vi "Save VI.vi"(8 "error in (no error)":errorcluster, 10 "Ctl Properties":T1[](array[typedef]), 11 "VI Properties":T2) -> (0 "error out":errorcluster, 2 "Status":bool, 3 "VI out":refnum<vi>)   [LabVIEW 2023, in "VI Properties Editor.lvlib"]
uses:
  VI Properties Editor.lvlib
  VI Properties.ctl
  <vilib>/picture/picture.llb/imagedata.ctl
  Control Properties.ctl
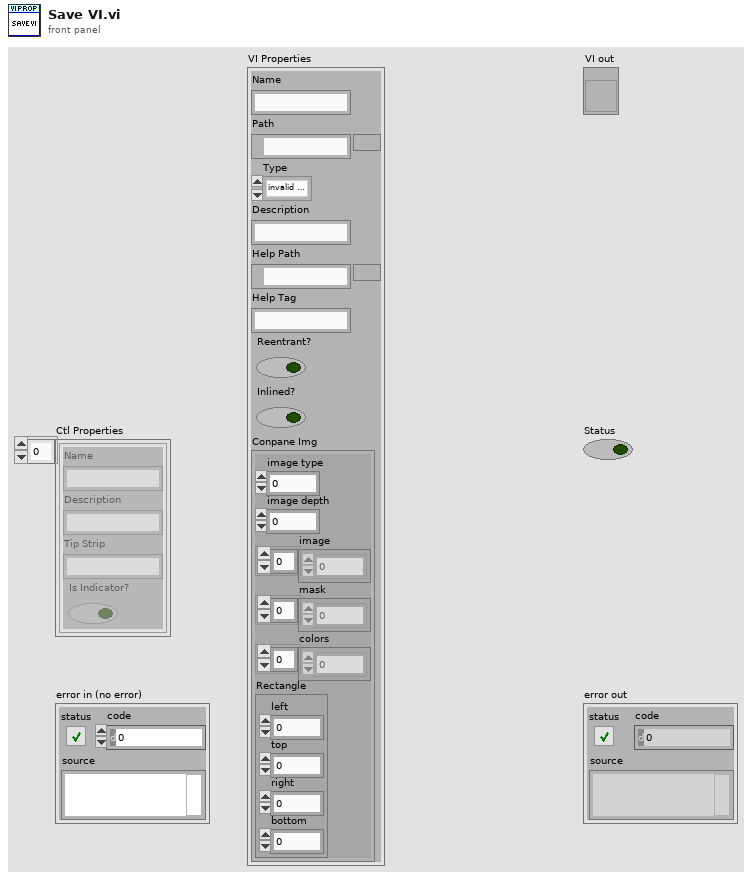
[diagram p1: front panel]
types:
  T1 = typedef "VI Properties Editor.lvlib/Control Properties.ctl" = cluster{"Name":string, "Description":string, "Tip Strip":string, "Is Indicator?":bool}
  T2 = typedef "VI Properties Editor.lvlib/VI Properties.ctl" = cluster{"Name":string, "Path":path, "Type":enum32{"invalid VI type", "Standard VI", "Control VI", "Global VI", "Polymorphic VI", "Configuration VI", "SubSystem", "Facade VI", "Method VI", "Statechart Diagram VI"}, "Description":string, "Help Path":path, "Help Tag":string, "Reentrant?":bool, "Inlined?":bool, "Conpane Img":T3}
  T3 = typedef "imagedata.ctl" = cluster{"image type":i32, "image depth":i32, "image":u8[], "mask":u8[], "colors":u32[], "Rectangle":cluster{"left":i16, "top":i16, "right":i16, "bottom":i16}}
  T4 = enum32{"invalid VI type", "Standard VI", "Control VI", "Global VI", "Polymorphic VI", "Configuration VI", "SubSystem", "Facade VI", "Method VI", "Statechart Diagram VI"}
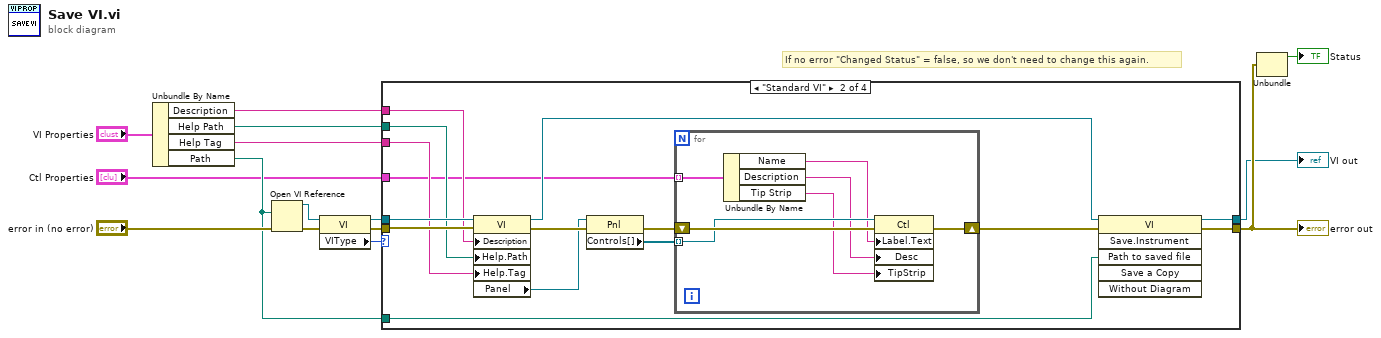
[diagram p0: block diagram]
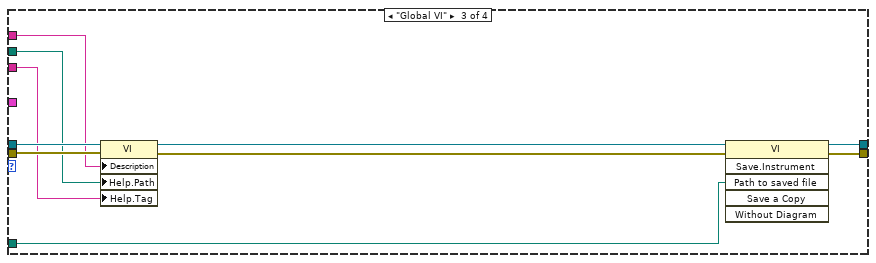
[diagram p3: hidden frame]
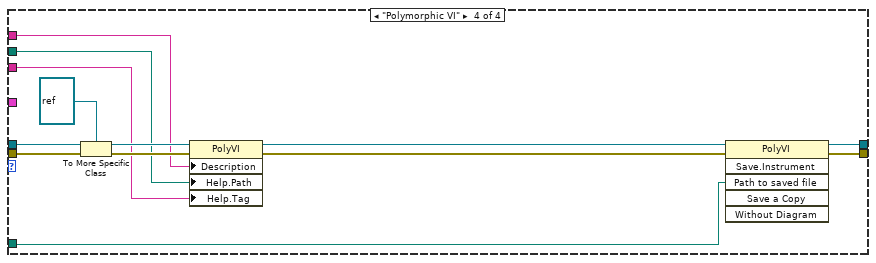
[diagram p4: hidden frame]
diagram:
  # "If no error \"Changed Status\" = false, so we don't need to change this again."
  n1 = Unbundle By Name("VI Properties") -> ("Description"=w3:string, "Help Path"=w2:path, "Help Tag"=w4:string, "Path"=w5:path)
  n2 = Open VI Reference(vi path=w5, error in (no error)="error in (no error)") -> (vi reference=w8:refnum<vi>, error out=w11:errorcluster)  [unwired: 4 in]
  n3 = property class="VI"(reference=w8, error in=w11) -> (reference out=w9:refnum<vi>, error out=w10:errorcluster, "VIType"=w12:T4)
  n4 = case shown="\"Standard VI\"" w12 {
    tunnel: [w16 w32 w49 w62] -> w13
    tunnel: [w17 w31 w48 w61] -> w14
    tunnel: w9 -> [w16 w23 w44 w58]
    tunnel: w10 -> [w17 w22 w43 w57]
    tunnel: w3 -> [_ w21 w40 w52]
    tunnel: w4 -> [_ w20 w42 w50]
    tunnel: w2 -> [_ w19 w41 w51]
    tunnel: w5 -> [_ w30 w47 w60]
    tunnel: "Ctl Properties" -> [_ w18 _ _]
    frame "invalid VI type", Default {
    }
    frame "Standard VI" {
      n5 = property class="VI"(reference=w23, error in=w22, "Description"=w21, "Help.Path"=w19, "Help.Tag"=w20) -> (reference out=w26:refnum<vi>, error out=w29:errorcluster, "Panel"=w28:refnum<vi>)
      n6 = property class="Pnl"(reference=w28, error in=w29) -> (error out=w24:errorcluster, "Controls[]"=w25:refnum<vi>[])  [unwired: 1 out]
      n7 = for {
        tunnel: w25 -> [w37] mode=indexing
        shift-right: [w39] -> w27
        shift-left: w24 -> [w38]
        tunnel: w18 -> [w36] mode=indexing
        n8 = Unbundle By Name(w36) -> ("Name"=w35:string, "Description"=w34:string, "Tip Strip"=w33:string)
        n9 = property class="Ctl"(reference=w37, error in=w38, "Label.Text"=w35, "Desc"=w34, "TipStrip"=w33) -> (error out=w39:errorcluster)  [unwired: 1 out]
      }
      n10 = invoke class="VI" method="Save.Instrument"(reference=w26, error in=w27, "Path to saved file"=w30) -> (reference out=w32:refnum<vi>, error out=w31:errorcluster)  [unwired: 3 in, 4 out]
    }
    frame "Global VI" {
      n11 = property class="VI"(reference=w44, error in=w43, "Description"=w40, "Help.Path"=w41, "Help.Tag"=w42) -> (reference out=w45:refnum<vi>, error out=w46:errorcluster)
      n12 = invoke class="VI" method="Save.Instrument"(reference=w45, error in=w46, "Path to saved file"=w47) -> (reference out=w49:refnum<vi>, error out=w48:errorcluster)  [unwired: 3 in, 4 out]
    }
    frame "Polymorphic VI" {
      n13 = To More Specific Class(target class=refnum<vi> refnum, reference=w58, error in=w57) -> (specific class reference=w56:refnum<vi>, error out=w55:errorcluster)
      n14 = property class="PolyVI"(reference=w56, error in=w55, "Description"=w52, "Help.Path"=w51, "Help.Tag"=w50) -> (reference out=w54:refnum<vi>, error out=w53:errorcluster)
      n15 = invoke class="PolyVI" method="Save.Instrument"(reference=w54, error in=w53, "Path to saved file"=w60) -> (reference out=w62:refnum<vi>, error out=w61:errorcluster)  [unwired: 3 in, 4 out]
    }
  }
  "error out" <- w14
  "VI out" <- w13
  n16 = Unbundle(w14) -> ("status"=→"Status":bool)  [unwired: 2 out]
